vi "Return to Middle.vi"(0 "handle":u32, 1 "Distance":sgl, 2 "Decel":sgl, 5 "Axis":i32, 7 "Sramp":sgl, 9 "Accel":sgl, 11 "error in (no error)":errorcluster caption="错误输入（无错误）", 12 "Lspeed":sgl, 13 "Speed":sgl) -> (4 "handle out":u32, 15 "error out":errorcluster caption="错误输出")   [LabVIEW 2015]
uses:
  zauxdll-2014/zauxdll.lvlib
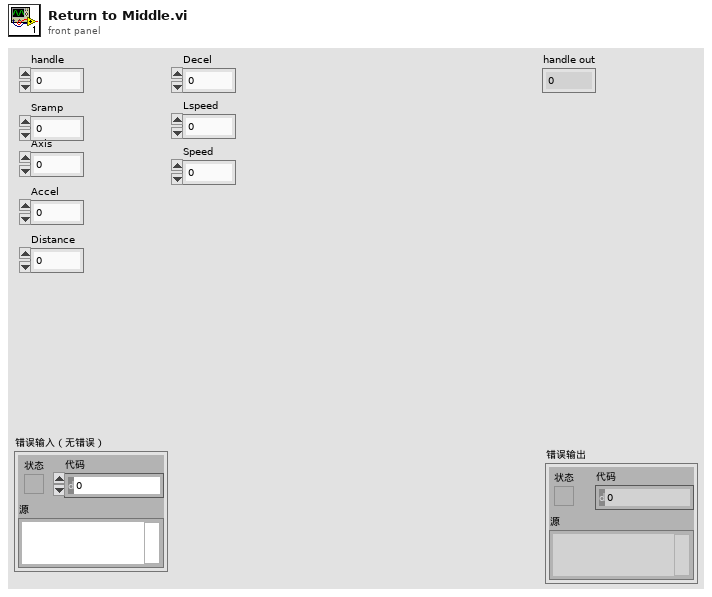
[diagram p1: front panel]
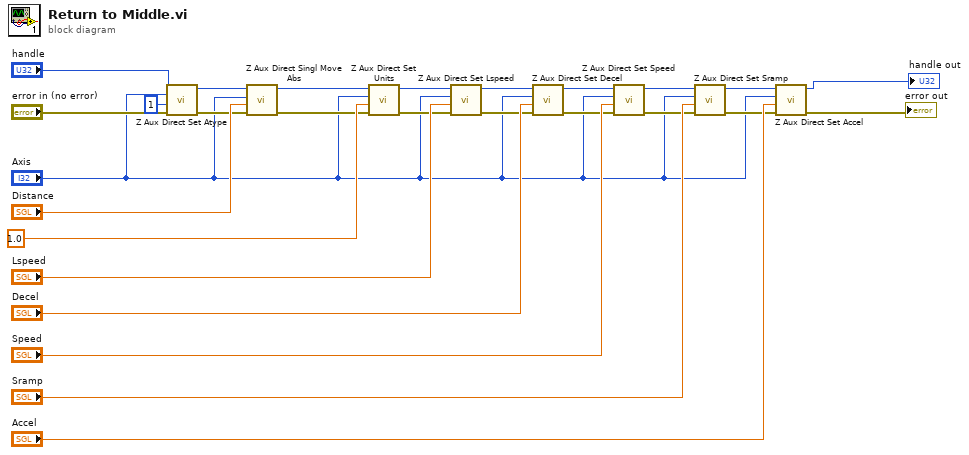
[diagram p0: block diagram]
diagram:
  n1 = call "Z Aux Direct Set Atype.vi"("error in (no error)"="error in (no error)", "iValue"=1, "iaxis"="Axis", "handle"="handle") -> ("error out"=w12:errorcluster, "handle out"=w26:u32)  [unwired: 5 in, 1 out]
  n2 = call "Z Aux Direct Singl Move Abs.vi"("error in (no error)"=w12, "fdistance"="Distance", "iaxis"="Axis", "handle"=w26) -> ("error out"=w11:errorcluster, "handle out"=w25:u32)  [unwired: 5 in, 1 out]
  n3 = call "Z Aux Direct Set Units.vi"("error in (no error)"=w11, "fValue"=sgl 1.0 ("Units"), "iaxis"="Axis", "handle"=w25) -> ("error out"=w6:errorcluster, "handle out"=w7:u32)  [unwired: 5 in, 1 out]
  n4 = call "Z Aux Direct Set Lspeed.vi"("error in (no error)"=w6, "fValue"="Lspeed", "iaxis"="Axis", "handle"=w7) -> ("error out"=w5:errorcluster, "handle out"=w4:u32)  [unwired: 5 in, 1 out]
  n5 = call "Z Aux Direct Set Decel.vi"("error in (no error)"=w5, "fValue"="Decel", "iaxis"="Axis", "handle"=w4) -> ("error out"=w10:errorcluster, "handle out"=w24:u32)  [unwired: 5 in, 1 out]
  n6 = call "Z Aux Direct Set Speed.vi"("error in (no error)"=w10, "fValue"="Speed", "iaxis"="Axis", "handle"=w24) -> ("error out"=w9:errorcluster, "handle out"=w23:u32)  [unwired: 5 in, 1 out]
  n7 = call "Z Aux Direct Set Sramp.vi"("error in (no error)"=w9, "fValue"="Sramp", "iaxis"="Axis", "handle"=w23) -> ("error out"=w8:errorcluster, "handle out"=w22:u32)  [unwired: 5 in, 1 out]
  n8 = call "Z Aux Direct Set Accel.vi"("error in (no error)"=w8, "fValue"="Accel", "iaxis"="Axis", "handle"=w22) -> ("error out"=→"error out":errorcluster, "handle out"=→"handle out":u32)  [unwired: 5 in, 1 out]
